vi "export_DFD.vi"(11 "index":i32) -> ()   [LabVIEW 2012]
uses:
  FT_HMI.llb/GLOBAL_PUMPS_PARAMS.vi
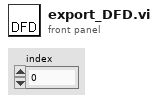
[diagram p1: front panel]
types:
  T1 = cluster{"VAC":cluster{"ENABLE":bool, "PUMPING_TIME [ms]":dbl, "MEASUREMENT_TIME [ms]":dbl, "PRESSURE_LIMIT [bar]":sgl}, "Q1":cluster{"ENABLE":bool, "PUMPING_TIME  [ms]":dbl, "MEASUREMENT_TIME  [ms]":sgl, "FLOW_TARGET  [ml/min]":sgl, "FLOW_LIMIT_UP  [ml/min]":sgl, "FLOW_LIMIT_DOWN [ml/min]":sgl, "PRESSURE_TARGET [bar]":sgl, "PRESSURE_LIMIT_UP [bar]":sgl, "PRESSURE_LIMIT_DOWN [bar]":sgl, "MAX_FLOW":bool}, "Q2":cluster{"ENABLE":bool, "PUMPING_TIME [ms]":dbl, "MEASUREMENT_TIME [ms]":dbl, "FLOW_TARGET [ml/min]":sgl, "FLOW_LIMIT_UP [ml/min]":sgl, "FLOW_LIMIT_DOWN [ml/min]":sgl, "PRESSURE_TARGET [bar]":sgl, "PRESSURE_LIMIT_UP [bar]":sgl, "PRESSURE_LIMIT_DOWN [bar]":sgl, "MAX_FLOW":bool}, "PMAX":cluster{"ENABLE":bool, "PUMPING_TIME [ms]":dbl, "MEASUREMENT_TIME [ms]":dbl, "PRESSURE_LIMIT [bar]":sgl, "PRESSURE_LOOSE_TIME [ms]":sgl}, "PRINT":cluster{"ENABLE":bool}, "SUPPLY":cluster{"VOLTAGE [V]":dbl, "FREQUENCY [Hz]":dbl}}
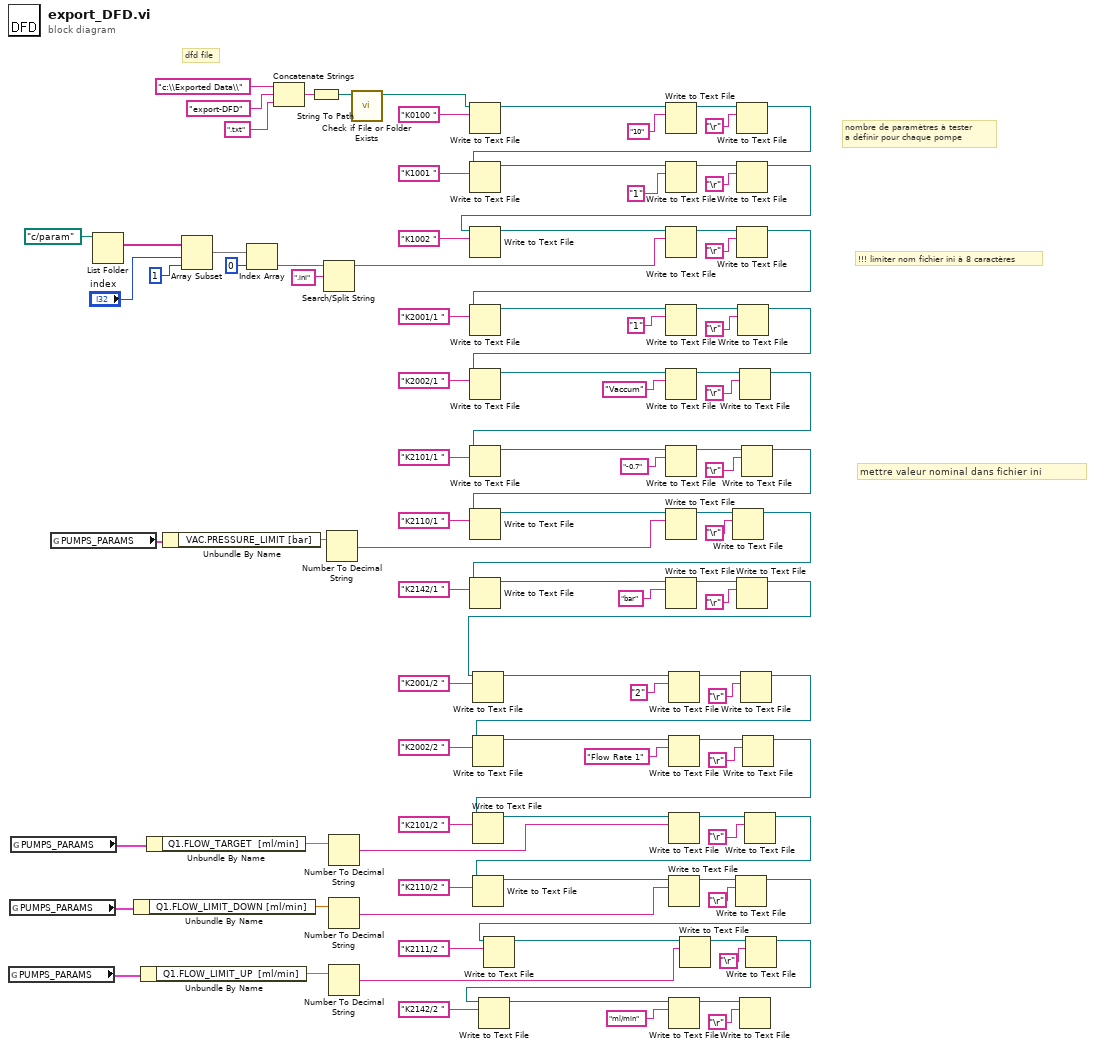
[diagram p0: block diagram]
diagram:
  # "dfd file"
  # "!!! limiter nom fichier ini à 8 caractères"
  # "nombre de paramètres à tester\na définir pour chaque pompe"
  # "mettre valeur nominal dans fichier ini"
  n1 = global read "GLOBAL_PUMPS_PARAMS.vi" "PUMPS_PARAMS"() -> (w10:T1)
  n2 = global read "GLOBAL_PUMPS_PARAMS.vi" "PUMPS_PARAMS"() -> (w42:T1)
  n3 = global read "GLOBAL_PUMPS_PARAMS.vi" "PUMPS_PARAMS"() -> (w13:T1)
  n4 = global read "GLOBAL_PUMPS_PARAMS.vi" "PUMPS_PARAMS"() -> (w83:T1)
  n5 = List Folder(path=path "c:/param") -> (filenames=w81:string[])  [unwired: 3 in, 3 out]
  n6 = Unbundle By Name(w42) -> ("Q1.FLOW_LIMIT_DOWN [ml/min]"=w20:sgl)
  n7 = Unbundle By Name(w10) -> ("Q1.FLOW_LIMIT_UP  [ml/min]"=w9:sgl)
  n8 = Unbundle By Name(w13) -> ("Q1.FLOW_TARGET  [ml/min]"=w12:sgl)
  n9 = Unbundle By Name(w83) -> ("VAC.PRESSURE_LIMIT [bar]"=w50:sgl)
  n10 = Array Subset(array=w81, index="index", length=1) -> (w74:string[])
  n11 = Index Array(array=w74, index=0) -> (element=w62:string)
  n12 = Concatenate Strings("c:\\Exported Data\\", "export-DFD" ("string"), ".txt") -> (w102:string)
  n13 = String To Path(string=w102) -> (path=w104:path)
  n14 = Search/Split String(string=w62, search string/char (-)=".ini") -> (substring before match=w64:string)  [unwired: 1 in, 2 out]
  n15 = Number To Decimal String(number=w50) -> (decimal integer string=w49:string)  [unwired: 1 in]
  n16 = Number To Decimal String(number=w12) -> (decimal integer string=w11:string)  [unwired: 1 in]
  n17 = Number To Decimal String(number=w20) -> (decimal integer string=w19:string)  [unwired: 1 in]
  n18 = Number To Decimal String(number=w9) -> (decimal integer string=w4:string)  [unwired: 1 in]
  n19 = call <vilib>:"Check if File or Folder Exists.vi"("path"=w104) -> ("dup path"=w99:path)  [unwired: 8 in, 2 out]
  n20 = Write to Text File(file (use dialog)=w99, text="K0100 ") -> (refnum out=w97:refnum<file>)  [unwired: 2 in, 2 out]
  n21 = Write to Text File(file (use dialog)=w97, text="10") -> (refnum out=w96:refnum<file>)  [unwired: 2 in, 2 out]
  n22 = Write to Text File(file (use dialog)=w96, text="\r") -> (refnum out=w89:refnum<file>)  [unwired: 2 in, 2 out]
  n23 = Write to Text File(file (use dialog)=w89, text="K1001 ") -> (refnum out=w92:refnum<file>)  [unwired: 2 in, 2 out]
  n24 = Write to Text File(file (use dialog)=w92, text="1") -> (refnum out=w91:refnum<file>)  [unwired: 2 in, 2 out]
  n25 = Write to Text File(file (use dialog)=w91, text="\r") -> (refnum out=w84:refnum<file>)  [unwired: 2 in, 2 out]
  n26 = Write to Text File(file (use dialog)=w84, text="K1002 ") -> (refnum out=w87:refnum<file>)  [unwired: 2 in, 2 out]
  n27 = Write to Text File(file (use dialog)=w87, text=w64) -> (refnum out=w86:refnum<file>)  [unwired: 2 in, 2 out]
  n28 = Write to Text File(file (use dialog)=w86, text="\r") -> (refnum out=w76:refnum<file>)  [unwired: 2 in, 2 out]
  n29 = Write to Text File(file (use dialog)=w76, text="K2001/1 ") -> (refnum out=w79:refnum<file>)  [unwired: 2 in, 2 out]
  n30 = Write to Text File(file (use dialog)=w79, text="1") -> (refnum out=w78:refnum<file>)  [unwired: 2 in, 2 out]
  n31 = Write to Text File(file (use dialog)=w78, text="\r") -> (refnum out=w66:refnum<file>)  [unwired: 2 in, 2 out]
  n32 = Write to Text File(file (use dialog)=w66, text="K2002/1 ") -> (refnum out=w70:refnum<file>)  [unwired: 2 in, 2 out]
  n33 = Write to Text File(file (use dialog)=w70, text="Vaccum") -> (refnum out=w69:refnum<file>)  [unwired: 2 in, 2 out]
  n34 = Write to Text File(file (use dialog)=w69, text="\r") -> (refnum out=w52:refnum<file>)  [unwired: 2 in, 2 out]
  n35 = Write to Text File(file (use dialog)=w52, text="K2101/1 ") -> (refnum out=w60:refnum<file>)  [unwired: 2 in, 2 out]
  n36 = Write to Text File(file (use dialog)=w60, text="-0.7") -> (refnum out=w59:refnum<file>)  [unwired: 2 in, 2 out]
  n37 = Write to Text File(file (use dialog)=w59, text="\r") -> (refnum out=w51:refnum<file>)  [unwired: 2 in, 2 out]
  n38 = Write to Text File(file (use dialog)=w51, text="K2110/1 ") -> (refnum out=w55:refnum<file>)  [unwired: 2 in, 2 out]
  n39 = Write to Text File(file (use dialog)=w55, text=w49) -> (refnum out=w54:refnum<file>)  [unwired: 2 in, 2 out]
  n40 = Write to Text File(file (use dialog)=w54, text="\r") -> (refnum out=w43:refnum<file>)  [unwired: 2 in, 2 out]
  n41 = Write to Text File(file (use dialog)=w43, text="K2142/1 ") -> (refnum out=w47:refnum<file>)  [unwired: 2 in, 2 out]
  n42 = Write to Text File(file (use dialog)=w47, text="bar") -> (refnum out=w46:refnum<file>)  [unwired: 2 in, 2 out]
  n43 = Write to Text File(file (use dialog)=w46, text="\r") -> (refnum out=w1:refnum<file>)  [unwired: 2 in, 2 out]
  n44 = Write to Text File(file (use dialog)=w1, text="K2001/2 ") -> (refnum out=w40:refnum<file>)  [unwired: 2 in, 2 out]
  n45 = Write to Text File(file (use dialog)=w40, text="2") -> (refnum out=w39:refnum<file>)  [unwired: 2 in, 2 out]
  n46 = Write to Text File(file (use dialog)=w39, text="\r") -> (refnum out=w31:refnum<file>)  [unwired: 2 in, 2 out]
  n47 = Write to Text File(file (use dialog)=w31, text="K2002/2 ") -> (refnum out=w35:refnum<file>)  [unwired: 2 in, 2 out]
  n48 = Write to Text File(file (use dialog)=w35, text="Flow Rate 1") -> (refnum out=w34:refnum<file>)  [unwired: 2 in, 2 out]
  n49 = Write to Text File(file (use dialog)=w34, text="\r") -> (refnum out=w22:refnum<file>)  [unwired: 2 in, 2 out]
  n50 = Write to Text File(file (use dialog)=w22, text="K2101/2 ") -> (refnum out=w29:refnum<file>)  [unwired: 2 in, 2 out]
  n51 = Write to Text File(file (use dialog)=w29, text=w11) -> (refnum out=w28:refnum<file>)  [unwired: 2 in, 2 out]
  n52 = Write to Text File(file (use dialog)=w28, text="\r") -> (refnum out=w21:refnum<file>)  [unwired: 2 in, 2 out]
  n53 = Write to Text File(file (use dialog)=w21, text="K2110/2 ") -> (refnum out=w25:refnum<file>)  [unwired: 2 in, 2 out]
  n54 = Write to Text File(file (use dialog)=w25, text=w19) -> (refnum out=w24:refnum<file>)  [unwired: 2 in, 2 out]
  n55 = Write to Text File(file (use dialog)=w24, text="\r") -> (refnum out=w3:refnum<file>)  [unwired: 2 in, 2 out]
  n56 = Write to Text File(file (use dialog)=w3, text="K2111/2 ") -> (refnum out=w7:refnum<file>)  [unwired: 2 in, 2 out]
  n57 = Write to Text File(file (use dialog)=w7, text=w4) -> (refnum out=w6:refnum<file>)  [unwired: 2 in, 2 out]
  n58 = Write to Text File(file (use dialog)=w6, text="\r") -> (refnum out=w2:refnum<file>)  [unwired: 2 in, 2 out]
  n59 = Write to Text File(file (use dialog)=w2, text="K2142/2 ") -> (refnum out=w17:refnum<file>)  [unwired: 2 in, 2 out]
  n60 = Write to Text File(file (use dialog)=w17, text="ml/min") -> (refnum out=w16:refnum<file>)  [unwired: 2 in, 2 out]
  n61 = Write to Text File(file (use dialog)=w16, text="\r") -> ()  [unwired: 2 in, 3 out]
